vi "getTrace_new.vi"(4 "에러 입력":errorcluster, 5 "ptr":u32, 6 "Refnum IN":refnum<file>, 7 "Trace attribute IN":T1) -> (0 "에러 출력":errorcluster, 1 "1D array":sgl[](array[numeric]), 2 "refnum OUT":refnum<file>, 3 "Trace attribute OUT":T1)   [LabVIEW 2017, in "HEKAdat.lvclass"]
uses:
  HEKAdat.lvclass
panel:
  out "Unit":string
  out "label":string
  out "nDatapoints":u32
  out "offset":u32
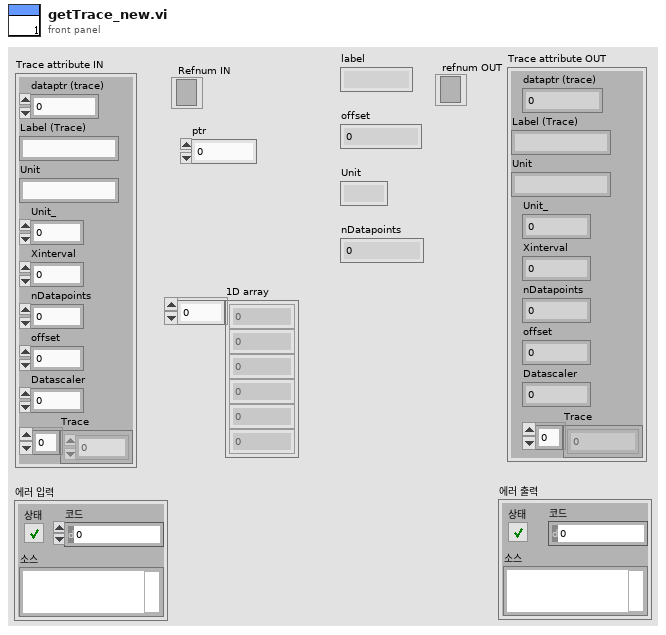
[diagram p1: front panel]
types:
  T1 = cluster{"dataptr (trace)":u32, "Label (Trace)":string, "Unit":string, "Unit_":dbl, "Xinterval":dbl, "nDatapoints":u32, "offset":u32, "Datascaler":dbl, "Trace":i16[]}
  T2 = enum16{"big-endian, network order", "native, host order", "little-endian"}
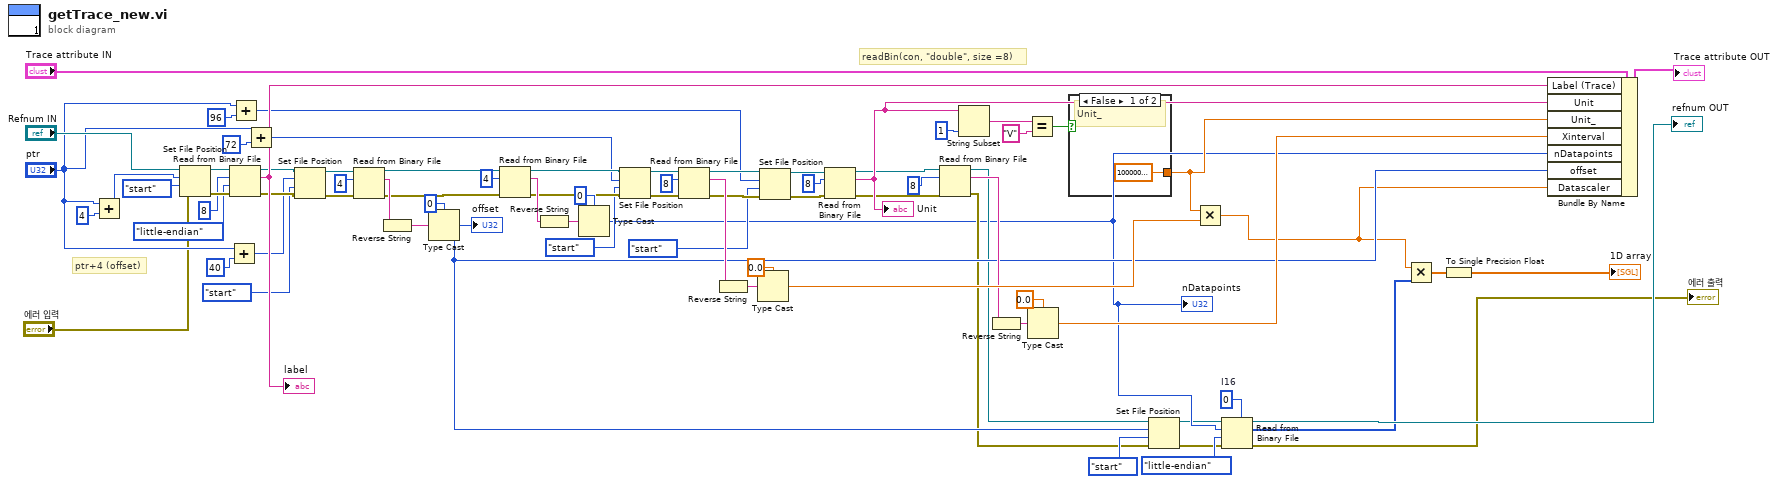
[diagram p0: block diagram]
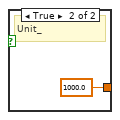
[diagram p2: hidden frame]
diagram:
  w8 = i16 0  # I16
  # "readBin(con, \"double\", size =8)"
  # "ptr+4 (offset)"
  n1 = Add(x="ptr", y=u32 4 ("length (rest)")) -> (x+y=w16:u32)
  n2 = Set File Position(offset (in bytes) (0)=w16, refnum="Refnum IN", from (0:start)=enum16{"start", "end", "current"}."start", error in="에러 입력") -> (refnum out=w54:refnum<file>, error out=w55:errorcluster)
  n3 = Add(x="ptr", y=u32 40 ("length (rest)")) -> (x+y=w48:u32)
  n4 = Read from Binary File(8:w55, 9:T2."little-endian" ("byte order (0:big-endian, network order)"), 10:u32 8 ("length (rest)"), 11:w54) -> (0:w50:errorcluster, 2:w51:string, 3:w49:refnum<file>)  [unwired: 2 in, 1 out]
  "label" <- w51
  n5 = Add(x="ptr", y=u32 96 ("length (rest)")) -> (x+y=w30:u32)
  n6 = Add(x="ptr", y=u32 72 ("length (rest)")) -> (x+y=w35:u32)
  n7 = Set File Position(offset (in bytes) (0)=w48, refnum=w49, from (0:start)=enum16{"start", "end", "current"}."start", error in=w50) -> (refnum out=w46:refnum<file>, error out=w47:errorcluster)
  n8 = Read from Binary File(8:w47, 10:u32 4 ("length (rest)"), 11:w46) -> (0:w43:errorcluster, 2:w44:string, 3:w42:refnum<file>)  [unwired: 3 in, 1 out]
  n9 = Reverse String(1:w44) -> (0:w63:string)
  n10 = Type Cast(type=u32 0, x=w63) -> (*(type *) &x=w21:u32)
  "offset" <- w21
  n11 = Read from Binary File(8:w43, 10:4 ("length (rest)"), 11:w42) -> (0:w36:errorcluster, 2:w40:string, 3:w37:refnum<file>)  [unwired: 3 in, 1 out]
  n12 = Reverse String(1:w40) -> (0:w67:string)
  n13 = Type Cast(type=u32 0, x=w67) -> (*(type *) &x=w5:u32)
  "nDatapoints" <- w5
  n14 = Set File Position(offset (in bytes) (0)=w35, refnum=w37, from (0:start)=enum16{"start", "end", "current"}."start", error in=w36) -> (refnum out=w38:refnum<file>, error out=w33:errorcluster)
  n15 = Read from Binary File(8:w33, 10:u32 8 ("length (rest)"), 11:w38) -> (0:w32:errorcluster, 2:w34:string, 3:w31:refnum<file>)  [unwired: 3 in, 1 out]
  n16 = Reverse String(1:w34) -> (0:w78:string)
  n17 = Type Cast(type=0.0, x=w78) -> (*(type *) &x=w58:dbl)
  n18 = Set File Position(offset (in bytes) (0)=w30, refnum=w31, from (0:start)=enum16{"start", "end", "current"}."start", error in=w32) -> (refnum out=w28:refnum<file>, error out=w29:errorcluster)
  n19 = Read from Binary File(8:w29, 10:u32 8 ("length (rest)"), 11:w28) -> (0:w25:errorcluster, 2:w26:string, 3:w24:refnum<file>)  [unwired: 3 in, 1 out]
  "Unit" <- w26
  n20 = Read from Binary File(8:w25, 10:u32 8 ("length (rest)"), 11:w24) -> (0:w12:errorcluster, 2:w22:string, 3:w13:refnum<file>)  [unwired: 3 in, 1 out]
  n21 = String Subset(string=w26, length (rest)=1 ("length (rest)")) -> (substring=w74:string)  [unwired: 1 in]
  n22 = Reverse String(1:w22) -> (0:w69:string)
  n23 = Equal?(x=w74, y="V") -> (x = y?=w73:bool)
  n24 = Type Cast(type=0.0, x=w69) -> (*(type *) &x=w61:dbl)
  n25 = case shown="False" w73 {
    tunnel: [1000000000000.0 ("xinterval 2") 1000.0 ("xinterval 2")] -> w59
    frame False {
      # "Unit_"
    }
    frame True {
      # "Unit_"
    }
  }
  n26 = Set File Position(offset (in bytes) (0)=w21, refnum=w13, from (0:start)=enum16{"start", "end", "current"}."start", error in=w12) -> (refnum out=w4:refnum<file>, error out=w3:errorcluster)
  n27 = Multiply(x=w59, y=w58) -> (x*y=w11:dbl)
  n28 = Read from Binary File(5:w8, 8:w3, 9:T2."little-endian" ("바이트 순서(0:big-endian, network order)"), 10:w5, 11:w4) -> (0:→"에러 출력":errorcluster, 2:w6:i16[], 3:→"refnum OUT":refnum<file>)  [unwired: 1 in, 1 out]
  n29 = Multiply(x=w11, y=w6) -> (x*y=w10:dbl[])
  n30 = To Single Precision Float(number=w10) -> (single precision float=→"1D array":sgl[])
  n31 = Bundle By Name(cluster="Trace attribute IN", "Label (Trace)"=w51, "Unit"=w26, "Unit_"=w59, "Xinterval"=w61, "nDatapoints"=w5, "offset"=w21, "Datascaler"=w11) -> (→"Trace attribute OUT":T1)
